vi "禹山pH_获取温度和测量值.vi"(8 "error in (no error)":errorcluster caption="错误输入（无错误）", 11 "MB session in":refnum<class "MB_Master.lvclass">) -> (0 "error out":errorcluster caption="错误输出", 2 "输出值":cluster{"温度测量值":sgl, "ORP":sgl, "pH":sgl}, 3 "MB session out":refnum<class "MB_Master.lvclass">)   [LabVIEW 2016, in "斯坦道多参数.lvlib"]
uses:
  <vilib>/Plasmionique/MB Master/MB_Master/MB_Master.lvclass
  <vilib>/Plasmionique/MB Master/MB Master.lvlib
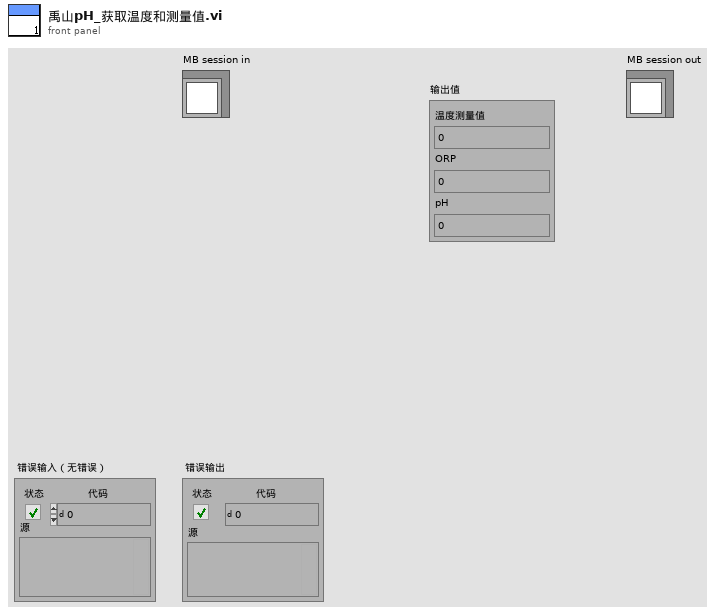
[diagram p1: front panel]
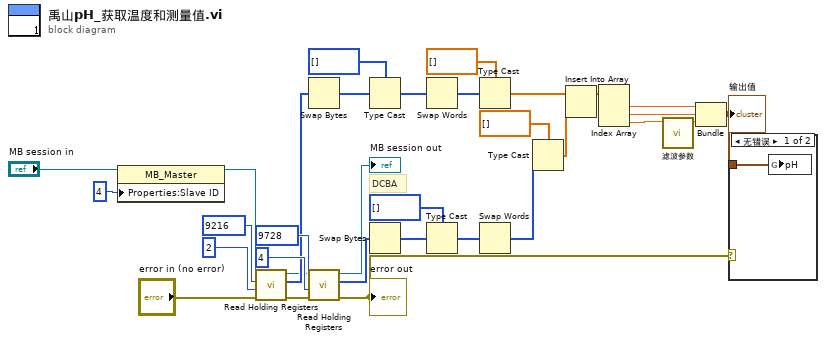
[diagram p0: block diagram]
diagram:
  # "DCBA"
  n1 = property class="MB_Master"(reference="MB session in", "Properties:Slave ID"=u16 4 ("y")) -> (reference out=w9:refnum<class "MB_Master.lvclass">)  [unwired: 1 in, 1 out]
  n2 = call <vilib>:"Read Holding Registers.vi"("error in (no error)"="error in (no error)", "quantity"=u16 2, "starting address"=u16 9216, "MB session in"=w9) -> ("error out"=w10:errorcluster, "Registers"=w13:u16[], "MB session out"=w8:refnum<class "MB_Master.lvclass">)  [unwired: 5 in]
  n3 = Swap Bytes(anything=w13) -> (byte swapped=w18:u16[])
  n4 = call <vilib>:"Read Holding Registers.vi"("error in (no error)"=w10, "quantity"=u16 4, "starting address"=u16 9728, "MB session in"=w8) -> ("error out"=w12:errorcluster, "Registers"=w25:u16[], "MB session out"=→"MB session out":refnum<class "MB_Master.lvclass">)  [unwired: 5 in]
  "error out" <- w12
  n5 = Type Cast(type=u32[] [] ("数组 2"), x=w18) -> (*(type *) &x=w16:u32[])
  n6 = Swap Bytes(anything=w25) -> (byte swapped=w24:u16[])
  n7 = Swap Words(1:w16) -> (0:w14:u32[])
  n8 = Type Cast(type=u32[] [] ("数组 2"), x=w24) -> (*(type *) &x=w28:u32[])
  n9 = Type Cast(type=sgl[] [] ("数组 2"), x=w14) -> (*(type *) &x=w7:sgl[])
  n10 = Swap Words(1:w28) -> (0:w30:u32[])
  n11 = Type Cast(type=sgl[] [] ("数组 2"), x=w30) -> (*(type *) &x=w5:sgl[])
  n12 = Insert Into Array(array=w7, new element=w5) -> (w6:sgl[])  [unwired: 1 in]
  n13 = Index Array(array=w6) -> (element #1=w23:sgl, element #2=w22:sgl, element #3=w2:sgl)  [unwired: 3 in]
  n14 = call "滤波参数.vi"("x"=w2) -> ("mode"=w1:dbl)  [unwired: 10 in]
  n15 = Bundle("数值"=w23, "数值"=w22, "mode"=w1) -> (w21:cluster{"数值":sgl, "数值":sgl, "mode":dbl})  [unwired: 1 in]
  "输出值" <- w21
  n16 = case shown="无错误" w12 {
    tunnel: w21 -> [w33 _]
    frame No Error {
      n17 = global write "禹山过程全局变量.vi" "pH"(w33) -> ()
    }
    frame Error {
    }
  }
